vi "TSM Scope Initialize Sessions.vi"(0 "TSM context":T1) -> (15 "error out":errorcluster)   [LabVIEW 2019]
doc: "Use this VI to initialize sessions for all NI-SCOPE instruments in the pin map associated with the test program."
uses:
  <vilib>/NI_TestStand_SemiconductorModule/NI_TestStand_Semiconductor_Module.lvlibp/PinMap/General/SemiconductorModuleContext.ctl
  <vilib>/NI_TestStand_SemiconductorModule/NI_TestStand_Semiconductor_Module.lvlibp
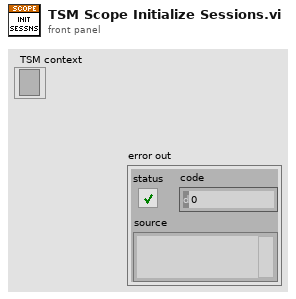
[diagram p1: front panel]
types:
  T1 = typedef "NI_TestStand_Semiconductor_Module.lvlibp/SemiconductorModuleContext.ctl" = refnum<k7>
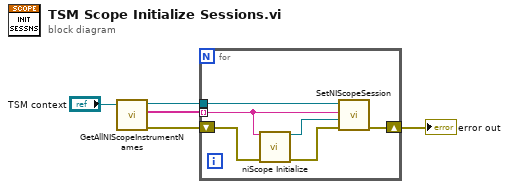
[diagram p0: block diagram]
diagram:
  n1 = call <vilib>:"GetAllNIScopeInstrumentNames.vi"("Semiconductor Module Context"="TSM context") -> ("error out"=w2:errorcluster, "Instrument Names"=w5:string[], "Semiconductor Module Context Out"=w4:T1)  [unwired: 8 in]
  n2 = for {
    tunnel: w5 -> [w9] mode=indexing
    tunnel: w4 -> [w6]
    shift-right: [w7] -> w1
    shift-left: w2 -> [w11]
    n3 = call <instrlib>:"niScope Initialize.vi"("resource name"=w9, "error in"=w11) -> ("instrument handle"=w8:refnum<k15>, "error out"=w10:errorcluster)  [unwired: 12 in]
    n4 = call <vilib>:"SetNIScopeSession.vi"("error in (no error)"=w10, "Instrument Session"=w8, "Instrument Name"=w9, "Semiconductor Module Context"=w6) -> ("error out"=w7:errorcluster)  [unwired: 6 in, 1 out]
  }
  "error out" <- w1
